vi "_Create.vi"(7 "Start Time Stamp":timestamp, 8 "Error In":errorcluster, 11 "Base Log Folder":path) -> (0 "Error Out":errorcluster, 3 "Log Out":refnum<file>)   [LabVIEW 2014, in "CF-Logger.lvlib"]
uses:
  CF-Logger.lvlib
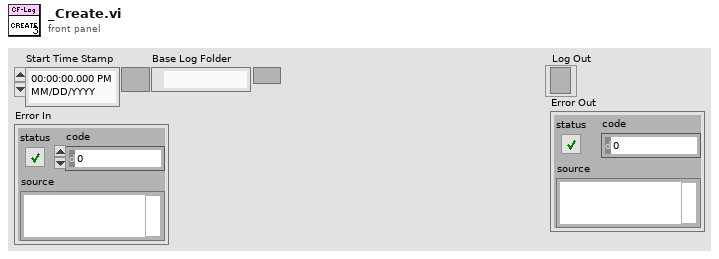
[diagram p1: front panel]
types:
  T1 = enum16{"open", "replace", "create", "open or create", "replace or create", "replace or create with confirmation"}
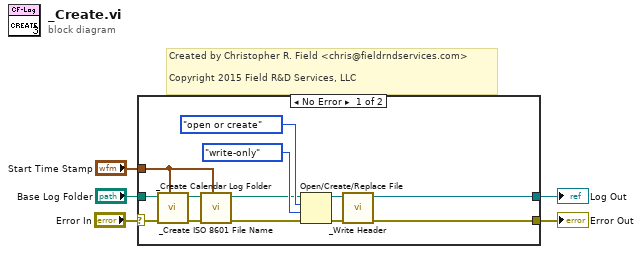
[diagram p0: block diagram]
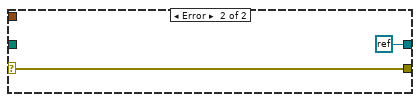
[diagram p2: hidden frame]
diagram:
  # "Created by Christopher R. Field <chris@fieldrndservices.com>\n\nCopyright 2015 Field R&D Services, LLC"
  n1 = case shown="No Error" "Error In" {
    selector: "Error In" -> [w15 w20]
    tunnel: "Base Log Folder" -> [w16 _]
    tunnel: "Start Time Stamp" -> [w12 _]
    tunnel: [w7 refnum<k0> refnum] -> w2
    tunnel: [w6 w20] -> w1
    frame No Error {
      n2 = call "_Create Calendar Log Folder.vi"("Start Time Stamp"=w12, "Error In"=w15, "Base Log Folder"=w16) -> ("Error Out"=w13:errorcluster, "Calendar Log Folder"=w14:path)  [unwired: 7 in]
      n3 = call "_Create ISO 8601 File Name.vi"("Start Time Stamp"=w12, "Error In"=w13, "Log Folder"=w14) -> ("Error Out"=w10:errorcluster, "ISO 8601 File"=w11:path)  [unwired: 7 in]
      n4 = Open/Create/Replace File(file path (use dialog)=w11, error in=w10, operation (0:open)=T1."open or create", access (0:read/write)=enum16{"read/write", "read-only", "write-only"}."write-only") -> (refnum out=w9:refnum<file>, error out=w8:errorcluster)  [unwired: 2 in, 1 out]
      n5 = call "_Write Header.vi"("Error In"=w8, "Log In"=w9) -> ("Error Out"=w6:errorcluster, "Log Out"=w7:refnum<file>)  [unwired: 8 in]
    }
    frame Error {
    }
  }
  "Log Out" <- w2
  "Error Out" <- w1
